vi "Reserve (N Sessions).vi"(6 "timeout in milliseconds":i32, 8 "error in":errorcluster, 9 "instrument type ID":string, 10 "pin or relay names":string[](array[string]), 11 "Measurement Context In":refnum<class "MeasurementContext.lvclass">) -> (0 "error out":errorcluster, 1 "gRPC channel pool out":T1, 2 "session information":T3[](array[typedef]), 3 "Measurement Context out":refnum<class "MeasurementContext.lvclass">)   [LabVIEW 2020, in "NIDCPowerSourceDCVoltage.lvlib"]
uses:
  NIDCPowerSourceDCVoltage.lvlib
  <vilib>/MeasurementLink/MeasurementLink Session Management Client/RPC Messages/ni_measurementlink_sessionmanagement_v1_SessionInformation.ctl
  <vilib>/MeasurementLink/MeasurementLink Session Management Client/RPC Messages/nidevice_grpc_Session.ctl
  <vilib>/MeasurementLink/MeasurementLink Session Management Client/RPC Messages/ni_measurementlink_sessionmanagement_v1_ChannelMapping.ctl
  GRPC Clients.ctl
  <vilib>/gRPC/LabVIEW gRPC Library/Shared/grpcId.ctl
  <vilib>/MeasurementLink/MeasurementLink Measurement Server/Classes/MeasurementContext/MeasurementContext.lvclass
  <vilib>/MeasurementLink/MeasurementLink Discovery Client/RPC Messages/ni_measurementlink_discovery_v1_ResolveServiceRequest.ctl
  <vilib>/MeasurementLink/MeasurementLink Session Management Client/RPC Messages/ni_measurementlink_sessionmanagement_v1_ReserveSessionsRequest.ctl
  <vilib>/MeasurementLink/MeasurementLink Session Management Client/RPC Messages/ni_measurementlink_PinMapContext.ctl
  <vilib>/MeasurementLink/MeasurementLink Measurement Server/MeasurementLink Measurement Server.lvlib
  <vilib>/MeasurementLink/MeasurementLink Discovery Client/MeasurementLink Discovery Client.lvlib
  <vilib>/MeasurementLink/MeasurementLink Session Management Client/MeasurementLink Session Management Client.lvlib
  <vilib>/gRPC/LabVIEW gRPC Library/grpc-lvsupport-release.lvlib
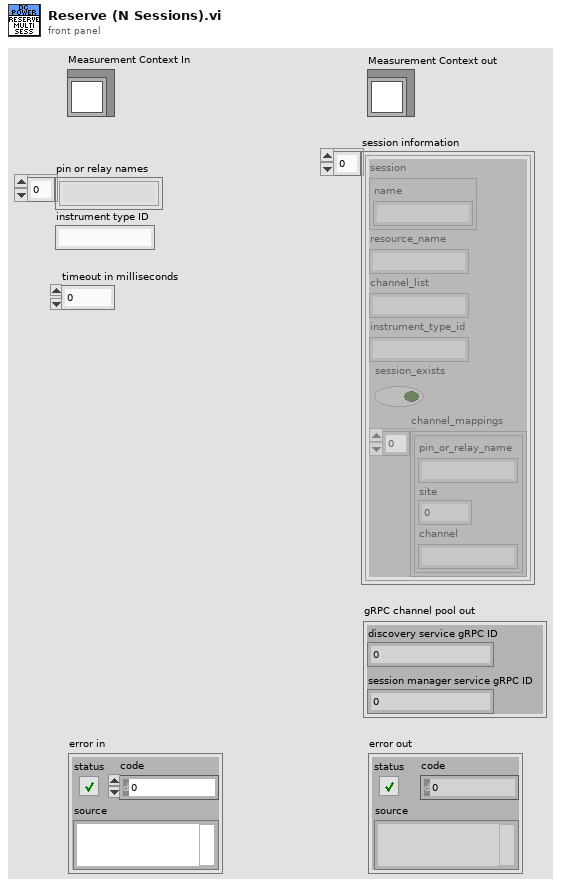
[diagram p1: front panel]
types:
  T1 = typedef "NIDCPowerSourceDCVoltage.lvlib/GRPC Clients.ctl" = cluster{"discovery service gRPC ID":T2, "session manager service gRPC ID":T2}
  T2 = typedef "grpc-lvsupport-release.lvlib/grpcId.ctl" = u64
  T3 = typedef "MeasurementLink Session Management Client.lvlib/ni_measurementlink_sessionmanagement_v1_SessionInformation.ctl" = cluster{"session":T4, "resource_name":string, "channel_list":string, "instrument_type_id":string, "session_exists":bool, "channel_mappings":T5[]}
  T4 = typedef "MeasurementLink Session Management Client.lvlib/nidevice_grpc_Session.ctl" = cluster{"name":string}
  T5 = typedef "MeasurementLink Session Management Client.lvlib/ni_measurementlink_sessionmanagement_v1_ChannelMapping.ctl" = cluster{"pin_or_relay_name":string, "site":i32, "channel":string}
  T6 = typedef "MeasurementLink Session Management Client.lvlib/ni_measurementlink_sessionmanagement_v1_ReserveSessionsRequest.ctl" = cluster{"pin_map_context":T7, "pin_or_relay_names":string[], "instrument_type_id":string, "timeout_in_milliseconds":i32}
  T7 = typedef "MeasurementLink Session Management Client.lvlib/ni_measurementlink_PinMapContext.ctl" = cluster{"pin_map_id":string, "sites":i32[]}
  T8 = typedef "MeasurementLink Discovery Client.lvlib/ni_measurementlink_discovery_v1_ResolveServiceRequest.ctl" = cluster{"provided_interface":string, "service_class":string}
  T9 = typedef "MeasurementLink Measurement Server.lvlib/PinMapContext.ctl" = cluster{"pin_map_id":string, "sites":i32[]}
  T10 = typedef "MeasurementLink Discovery Client.lvlib/ni_measurementlink_discovery_v1_ServiceLocation.ctl" = cluster{"location":string, "insecure_port":string, "ssl_authenticated_port":string}
  T11 = typedef "MeasurementLink Session Management Client.lvlib/ni_measurementlink_sessionmanagement_v1_ReserveSessionsResponse.ctl" = cluster{"sessions":T3[]}
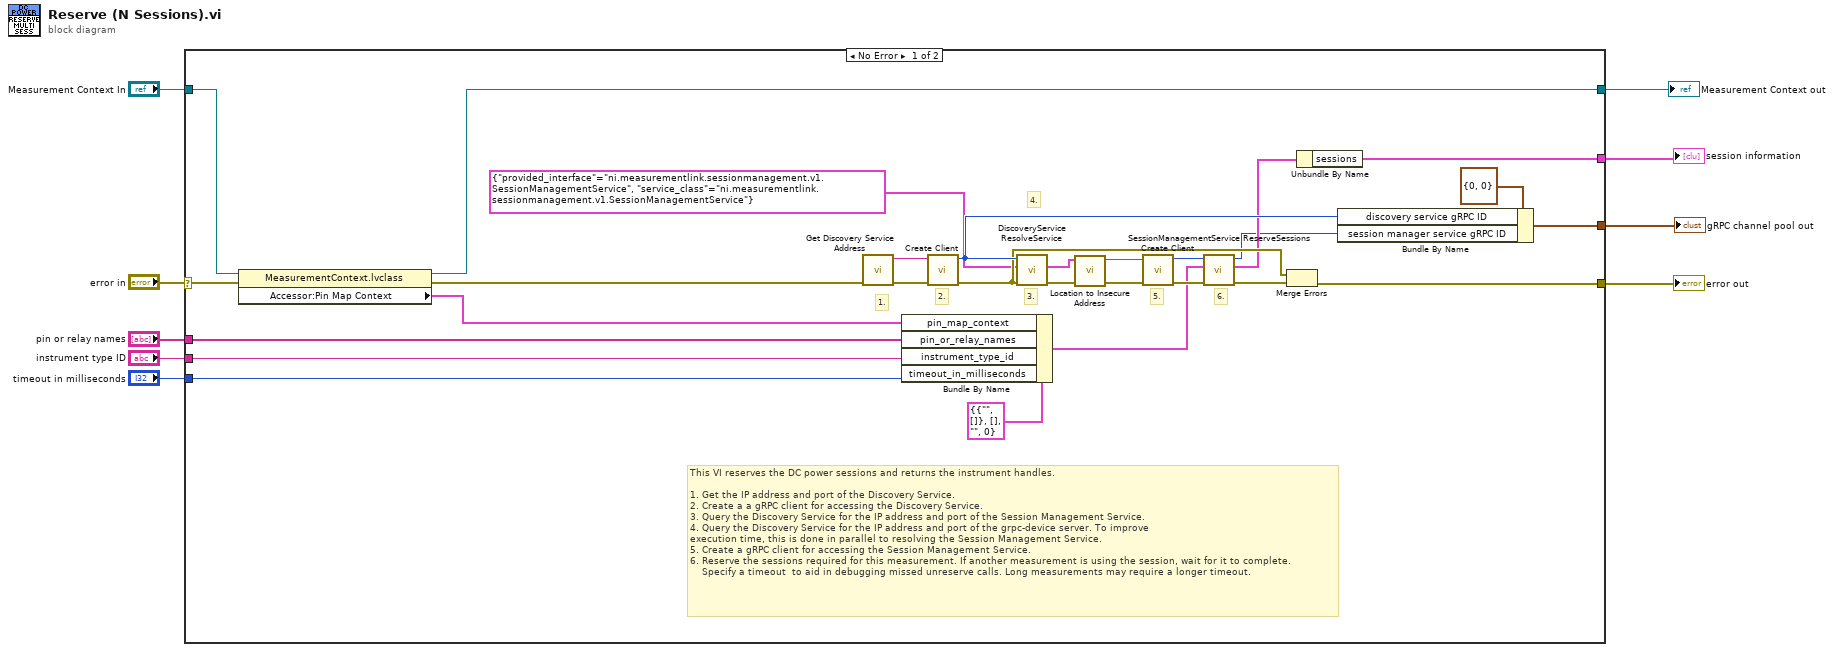
[diagram p0: block diagram]
diagram:
  n1 = case shown="No Error" "error in" {
    selector: "error in" -> [w10 w38]
    tunnel: [w26 w38] -> w9
    tunnel: "instrument type ID" -> [w24 _]
    tunnel: "timeout in milliseconds" -> [w23 _]
    tunnel: "pin or relay names" -> [w21 _]
    tunnel: [w20 _] -> w5
    tunnel: [w15 _] -> w4
    tunnel: "Measurement Context In" -> [w13 w37]
    tunnel: [w11 w37] -> w2
    frame No Error {
      # "6."
      # "5."
      # "4."
      # "3."
      # "2."
      # "1."
      # "This VI reserves the DC power sessions and returns the instrument handles.\n\n1. Get the IP address and port of the Discovery Service.\n2. Create a a gRPC client for accessing the Discovery Service.\n3. Query the Discovery Service for the IP address and port of the Session Management Service.\n4. Query the Discovery Service for the IP address and port of the grpc-device server. To improve \nexecution time, this is done in parallel to resolving the Session Management Service.\n5. Create a gRPC client for accessing the Session Management Service.\n6. Reserve the sessions required for this measurement. If another measurement is using the session, wait for it to complete. \n    Specify a timeout  to aid in debugging missed unreserve calls. Long measurements may require a longer timeout."
      n2 = property class="MeasurementContext.lvclass"(reference=w13, error in=w10) -> (reference out=w11:refnum<class "MeasurementContext.lvclass">, error out=w14:errorcluster, "Accessor:Pin Map Context"=w12:T9)
      n3 = call <vilib>:"Get Discovery Service Address.vi"("error in"=w14) -> ("error out"=w36:errorcluster, "address"=w35:string)  [unwired: 9 in]
      n4 = Bundle By Name(cluster=T6 {"pin_map_context"={"pin_map_id"="", "sites"=[]}, "pin_or_relay_names"=[], "instrument_type_id"="", "timeout_in_milliseconds"=0} ("Request Data"), "pin_map_context"=w12, "pin_or_relay_names"=w21, "instrument_type_id"=w24, "timeout_in_milliseconds"=w23) -> (w22:T6)
      n5 = call <vilib>:"Create Client.vi"("error in"=w36, "address"=w35) -> ("error out"=w29:errorcluster, "gRPC ID Out"=w30:T2)  [unwired: 8 in]
      n6 = call <vilib>:"DiscoveryService ResolveService.vi"("error in"=w29, "Request Data"=T8 {"provided_interface"="ni.measurementlink.sessionmanagement.v1.SessionManagementService", "service_class"="ni.measurementlink.sessionmanagement.v1.SessionManagementService"}, "gRPC ID"=w30) -> ("error out"=w32:errorcluster, "Response Data"=w19:T10)  [unwired: 6 in, 1 out]
      n7 = call "Location to Insecure Address.vi"("Response Data"=w19) -> ("String"=w18:string)  [unwired: 10 in]
      n8 = call <vilib>:"Create Client.vi"("error in"=w32, "address"=w18) -> ("error out"=w33:errorcluster, "gRPC ID Out"=w34:T2)  [unwired: 8 in]
      n9 = call <vilib>:"SessionManagementService ReserveSessions.vi"("error in"=w33, "Request Data"=w22, "gRPC ID"=w34) -> ("error out"=w31:errorcluster, "Response Data"=w27:T11, "gRPC ID out"=w17:T2)  [unwired: 6 in]
      n10 = Merge Errors(w29, w31) -> (w26:errorcluster)
      n11 = Unbundle By Name(w27) -> ("sessions"=w20:T3[])
      n12 = Bundle By Name(cluster=T1 {"discovery service gRPC ID"=0, "session manager service gRPC ID"=0} ("gRPC channel pool out"), "discovery service gRPC ID"=w30, "session manager service gRPC ID"=w17) -> (w15:T1)
    }
    frame Error {
    }
  }
  "error out" <- w9
  "session information" <- w5
  "gRPC channel pool out" <- w4
  "Measurement Context out" <- w2
